vi "Configure Operation.vi"(6 "Continous Mode Meas Rate":u8(ring) items=["1 Hz Meas Rate"=0, "5 Hz Meas Rate"=32, "10 Hz Meas Rate"=64, "20 Hz Meas Rate"=96], 7 "I2C Channel":u8, 8 "error in (no error)":errorcluster, 9 "Periodic Set/Reset":u8(ring)=16 items=["OFF"=0, "ON"=16], 10 "Operational Mode":u8(ring) items=["Standby Mode", "Query Mode", "Continuous Mode"], 11 "LINX Resource In":T1) -> (0 "error out":errorcluster, 3 "LINX Resource Out":T1)   [LabVIEW 2014, in "LMH-LINX.lvlib" / "HMC6352.lvlib"]
uses:
  <vilib>/MakerHub/LINX/Public/Sensors/Orientation/Compass/HMC6352/HMC6352.lvlib
  <vilib>/MakerHub/LINX/Private/Type Defs/LINX Ref.ctl
  <vilib>/MakerHub/LINX/Private/Type Defs/Platform.ctl
  <vilib>/MakerHub/LINX/Private/Type Defs/Interface.ctl
  <vilib>/MakerHub/LINX/Private/Device/Type Defs/LINX Device Config.ctl
  <vilib>/MakerHub/LINX/Private/Device/Type Defs/TCP Config.ctl
  <vilib>/MakerHub/LINX/Private/Device/Type Defs/Channels.ctl
  <vilib>/MakerHub/LINX/LMH-LINX.lvlib
  <vilib>/MakerHub/LINX/Private/Device/Device.lvlib
panel:
  # "INPUTS"
  # "OUTPUTS"
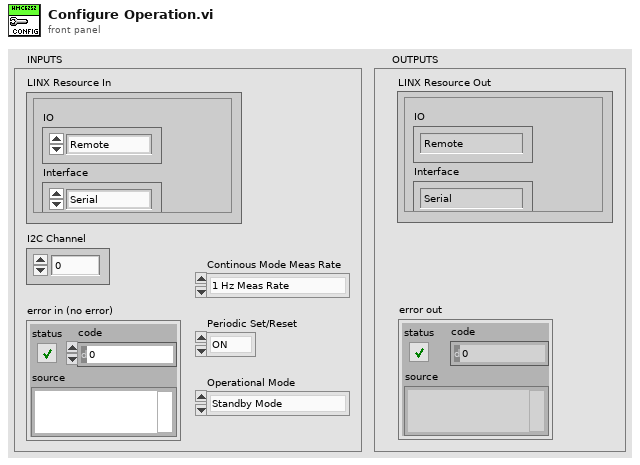
[diagram p1: front panel]
types:
  T1 = typedef "LMH-LINX.lvlib/LINX Ref.ctl" = cluster{"IO":T2, "Interface":T3, "LINX Device Config":T4}
  T2 = typedef "LMH-LINX.lvlib/Platform.ctl" = enum16{"Remote", "Local"}
  T3 = typedef "LMH-LINX.lvlib/Interface.ctl" = enum16{"Serial", "TCP"}
  T4 = typedef "LMH-LINX.lvlib/Device.lvlib/LINX Device Config.ctl" = cluster{"Interface":T3, "COM Port":refnum<visa-resource-name>, "TCP Configuration":T5, "Device Family":u8, "Device ID":u8, "Device Name":string, "TCP Ref":refnum<k5>, "Channels":T6}
  T5 = typedef "LMH-LINX.lvlib/Device.lvlib/TCP Config.ctl" = cluster{"IP Address":string, "Port":u16}
  T6 = typedef "LMH-LINX.lvlib/Channels.ctl" = cluster{"DI":u8[], "DO":u8[], "AI":u8[], "AO":u8[], "PWM":u8[], "QE":u8[], "UART":u8[], "I2C 2":u8[], "SPI":u8[], "CAN":u8[], "Servo":u8[], "AI Ref (V)":dbl, "AI Resolution (Bits)":u8, "AO Ref (V)":dbl, "AO Resolution (Bits)":u8}
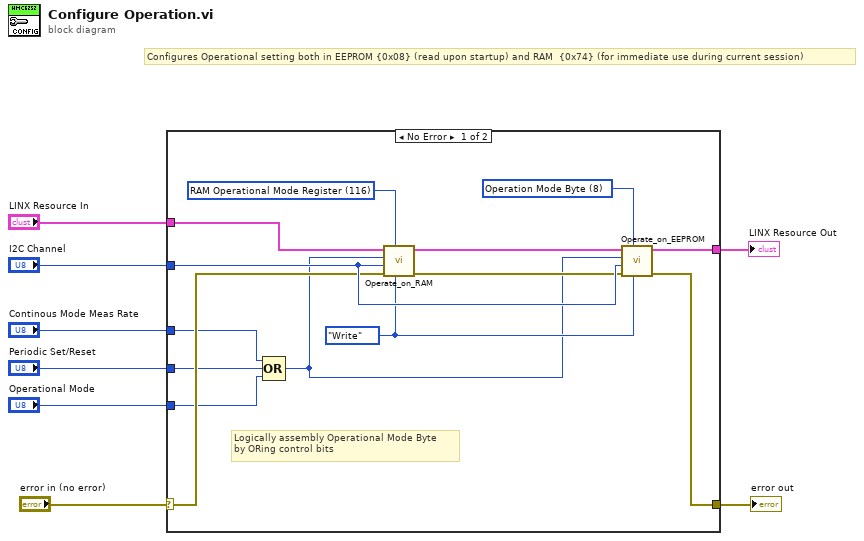
[diagram p0: block diagram]
diagram:
  # "Configures Operational setting both in EEPROM {0x08} (read upon startup) and RAM  {0x74} (for immediate use during current session)"
  n1 = case shown="No Error" "error in (no error)" {
    selector: "error in (no error)" -> [w14 w24]
    tunnel: [w20 w24] -> w7
    tunnel: "LINX Resource In" -> [w19 w23]
    tunnel: "I2C Channel" -> [w16 _]
    tunnel: [w21 w23] -> w4
    tunnel: "Operational Mode" -> [w10 _]
    tunnel: "Periodic Set/Reset" -> [w11 _]
    tunnel: "Continous Mode Meas Rate" -> [w12 _]
    frame No Error {
      w13 = enum16{"Write", "Read"}."Write" ("Operation")
      w17 = u8 116 items=["RAM Operational Mode Register"=116] ("RAM Registers Addresses")
      w22 = u8 8 items=["I2C Slave Address", "Magnetometer X Offset MSB", "Magnetometer X Offset LSB", "Magnetometer Y Offset MSB", "Magnetometer Y Offset LSB", "Measurement Time Delay", "Number of Summed Measurements", "Software Version Number", "Operation Mode Byte"] ("EEPROM Addresses")
      # "Logically assembly Operational Mode Byte\nby ORing control bits"
      n2 = Compound Arithmetic op=OR(w12, w11, w10) -> (w9:u8)
      n3 = call <vilib>:"Operate_on_RAM.vi"("Operation"=w13, "RAM Addresses"=w17, "error in (no error)"=w14, "I2C Channel"=w16, "Data"=w9, "LINX Resource In"=w19) -> ("error out"=w15:errorcluster, "LINX Resource Out"=w18:T1)  [unwired: 3 in, 1 out]
      n4 = call <vilib>:"Operate_on_EEPROM.vi"("Operation"=w13, "EEPROM Addresses"=w22, "error in (no error)"=w15, "I2C Channel"=w16, "Data"=w9, "LINX Resource In"=w18) -> ("error out"=w20:errorcluster, "LINX Resource Out"=w21:T1)  [unwired: 3 in, 1 out]
    }
    frame Error {
    }
  }
  "error out" <- w7
  "LINX Resource Out" <- w4
